vi "Pratik3-Case2.vi"() -> ()   [LabVIEW 2024]
panel:
  out "x/y 3":dbl
  in  "Dalga Frekansı(Hz)":dbl=40.0 min=40.0 step=1000000.0 format="%#_9g"
  out "MESSAGE":string
  out "lo(x)":u8 format="%x"
  out "hi(x)":u8 format="%x"
  out "x/y":dbl
  in  "Dalga Genliği(mV)":dbl min=0.0 max=376000.0 step=11.5
  out "Byte0":u32 format="%x"
  out "lo(x) 3":u8 format="%x"
  out "hi(x) 3":u8 format="%x"
  out "lo(x) 2":u8 format="%x"
  out "hi(x) 2":u8 format="%1x"
  out "x/y 2":dbl
  in  "Dalga Fazı(’C)":dbl min=0.0 max=360.0 step=1.0
  in  "Dalga Şekli":enum16{"Kare", "Üçgen", "Sinüs", "Testere Dişi"}(ring)
  # "High Byte: (12345/11,5) / 256 = 4 (0x04)"
  # "Low Byte: 1073 % 256 = 49 (0x31)"
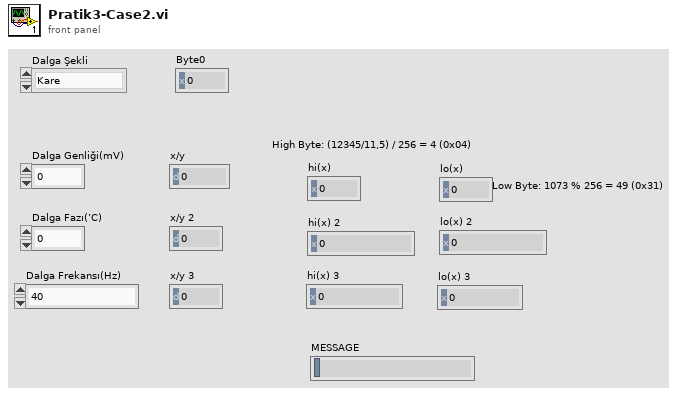
[diagram p1: front panel]
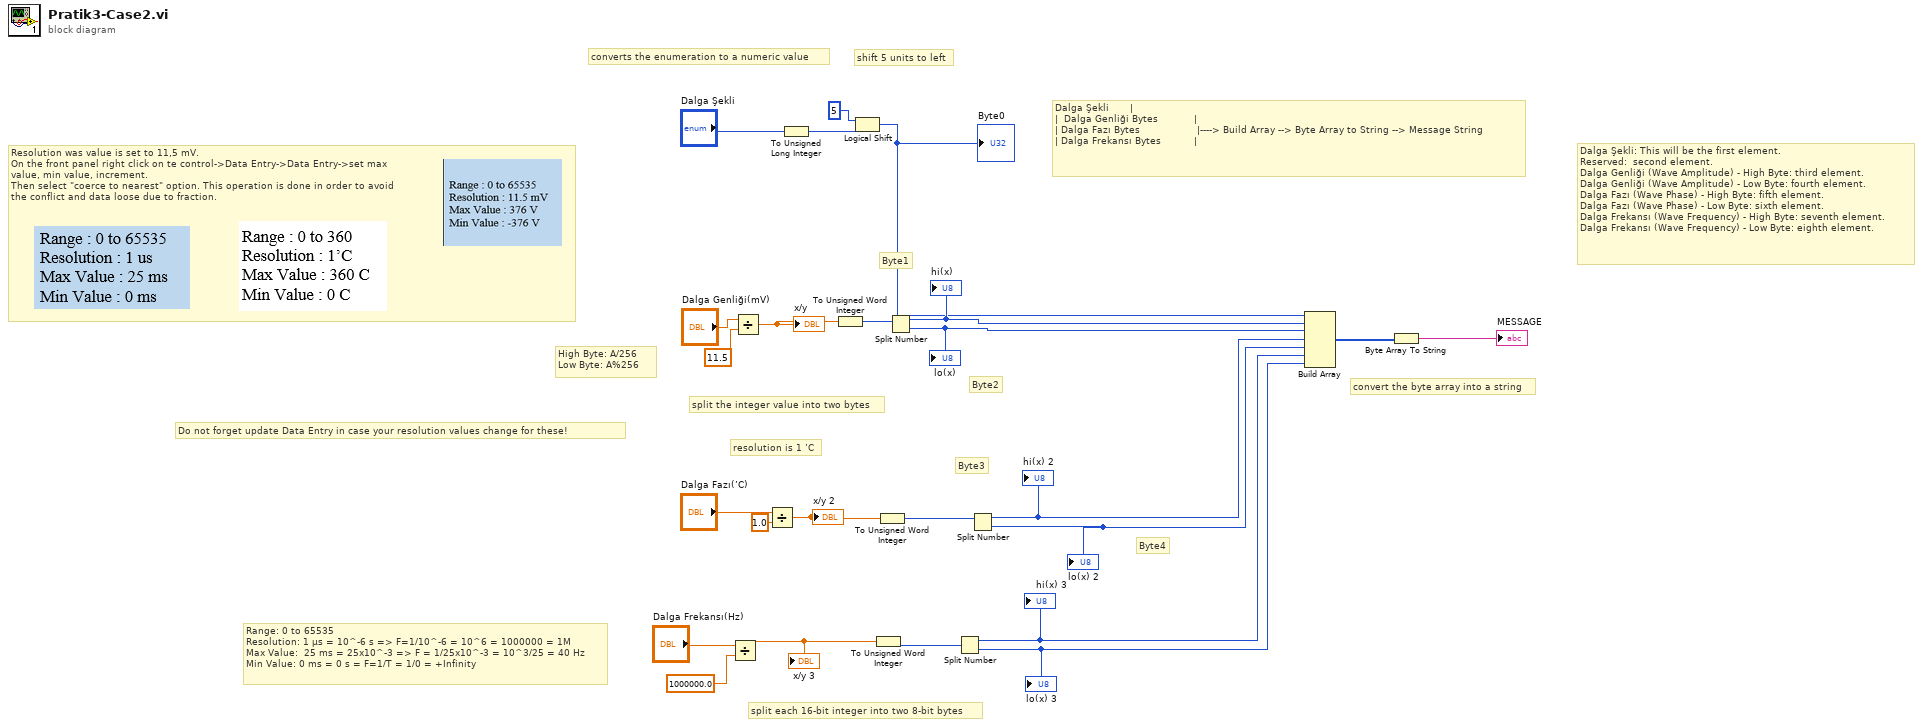
[diagram p0: block diagram]
diagram:
  # "Do not forget update Data Entry in case your resolution values change for these!"
  # "Range: 0 to 65535\nResolution: 1 µs = 10^-6 s => F=1/10^-6 = 10^6 = 1000000 = 1M\nMax Value:  25 ms = 25x10^-3 => F = 1/25x10^-3 = 10^3/25 = 40 Hz\nMin Value: 0 ms = 0 s = F=1/T = 1/0 = +Infinity"
  # "resolution is 1 ’C"
  # "Resolution was value is set to 11,5 mV.\nOn the front panel right click on te control->Data Entry->Data Entry->set max \nvalue, min value, increment.\nThen select \"coerce to nearest\" option. This operation is done in order to avoid \nthe conflict and data loose due to fraction."
  # "High Byte: A/256\nLow Byte: A%256"
  # "Dalga Şekli: This will be the first element.\nReserved:  second element.\nDalga Genliği (Wave Amplitude) - High Byte: third element.\nDalga Genliği (Wave Amplitude) - Low Byte: fourth element.\nDalga Fazı (Wave Phase) - High Byte: fifth element.\nDalga Fazı (Wave Phase) - Low Byte: sixth element.\nDalga Frekansı (Wave Frequency) - High Byte: seventh element.\nDalga Frekansı (Wave Frequency) - Low Byte: eighth element."
  # "Dalga Şekli       |\n|  Dalga Genliği Bytes            |        \n| Dalga Fazı Bytes                   |----> Build Array --> Byte Array to String --> Message String\n| Dalga Frekansı Bytes           |"
  # "convert the byte array into a string"
  # "split each 16-bit integer into two 8-bit bytes"
  # "split the integer value into two bytes"
  # "Byte4"
  # "Byte3"
  # "Byte2"
  # "Byte1"
  # "shift 5 units to left"
  # "converts the enumeration to a numeric value"
  n1 = Divide(x="Dalga Frekansı(Hz)", y=1000000.0) -> (x/y=w1:dbl)
  "x/y 3" <- w1
  n2 = Divide(x="Dalga Genliği(mV)", y=11.5) -> (x/y=w9:dbl)
  "x/y" <- w9
  n3 = Divide(x="Dalga Fazı(’C)", y=1.0) -> (x/y=w21:dbl)
  "x/y 2" <- w21
  n4 = To Unsigned Long Integer(number="Dalga Şekli") -> (unsigned 32bit integer=w17:u32)
  n5 = To Unsigned Word Integer(number=w9) -> (unsigned 16bit integer=w8:u16)
  n6 = Logical Shift(y=i16 5, x=w17) -> (x << y=w4:u32)
  "Byte0" <- w4
  n7 = To Unsigned Word Integer(number=w1) -> (unsigned 16bit integer=w19:u16)
  n8 = To Unsigned Word Integer(number=w21) -> (unsigned 16bit integer=w20:u16)
  n9 = Split Number(x=w8) -> (hi(x)=w7:u8, lo(x)=w6:u8)
  "hi(x)" <- w7
  "lo(x)" <- w6
  n10 = Split Number(x=w19) -> (hi(x)=w15:u8, lo(x)=w14:u8)
  "hi(x) 3" <- w15
  "lo(x) 3" <- w14
  n11 = Split Number(x=w20) -> (hi(x)=w13:u8, lo(x)=w16:u8)
  "hi(x) 2" <- w13
  "lo(x) 2" <- w16
  n12 = Build Array "Build Array"(w4, w7, w6, w13, w16, w15, w14) -> (w12:u32[])
  n13 = Byte Array To String(unsigned byte array=w12) -> (string=→"MESSAGE":string)
